vi "Set VI Under Test.vi"(8 "error in (no error)":errorcluster, 10 "VI Under Test Path":path, 11 "LUnit Test Vector In":refnum<class "LUnit Test Vector.lvclass">) -> (0 "error out":errorcluster, 3 "LUnit Test Vector Out":refnum<class "LUnit Test Vector.lvclass">)   [LabVIEW 2020, in "LUnit Test Vector.lvclass"]
doc: "Sets the VI under test. The VI specified is exercised when the Execute Test Vector VI is called."
uses:
  LUnit Test Vector.lvclass
  LUnit Test Vector.lvclass/LUnit Test Vector.ctl
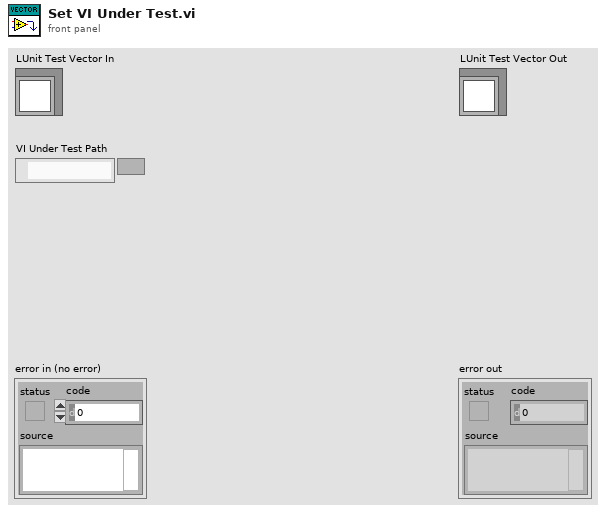
[diagram p1: front panel]
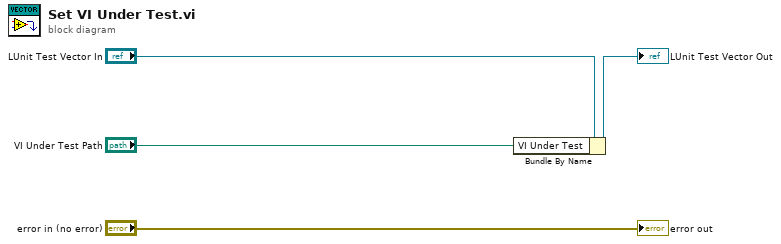
[diagram p0: block diagram]
diagram:
  n1 = Bundle By Name(cluster="LUnit Test Vector In", "VI Under Test"="VI Under Test Path") -> (→"LUnit Test Vector Out":refnum<class "LUnit Test Vector.lvclass">)
  "error out" <- "error in (no error)"
